vi "stop_sweep.vi"(8 "error in (no error)":errorcluster, 11 "Stimulator090724Scaffold in":refnum<class "Stimulator090724Scaffold.lvclass">) -> (0 "error out":errorcluster, 3 "Stimulator090724Scaffold out":refnum<class "Stimulator090724Scaffold.lvclass">)   [LabVIEW 2010, in "Stimulator090724Scaffold.lvclass"]
uses:
  Stimulator090724Scaffold.lvclass
  Stimulator090724Scaffold.lvclass/Stimulator090724Scaffold.ctl
  Clock/GenericClock/GenericClock/GenericClock.lvclass
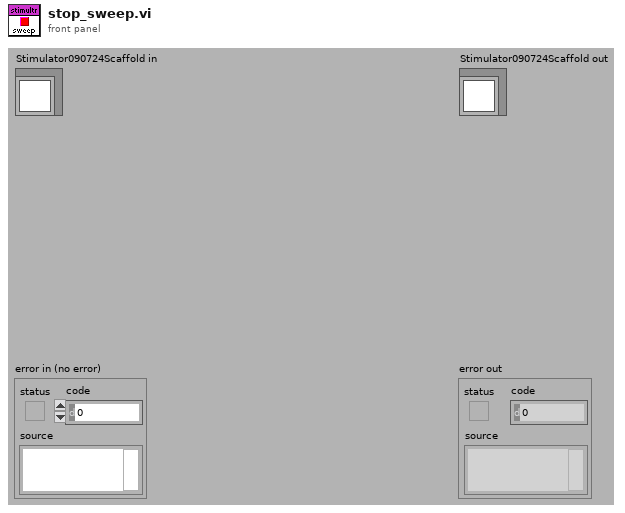
[diagram p1: front panel]
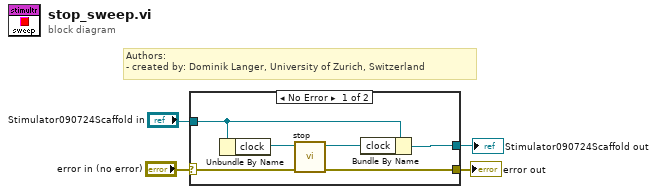
[diagram p0: block diagram]
diagram:
  # "Authors: \n- created by: Dominik Langer, University of Zurich, Switzerland"
  n1 = case shown="No Error" "error in (no error)" {
    selector: "error in (no error)" -> [w7 w12]
    tunnel: [w6 w12] -> w2
    tunnel: [w5 w11] -> w1
    tunnel: "Stimulator090724Scaffold in" -> [w9 w11]
    frame No Error {
      n2 = Unbundle By Name(w9) -> ("clock"=w10:refnum<class "GenericClock.lvclass">)
      n3 = call-dynamic "stop.vi"("error in (no error)"=w7, "GenericClock in"=w10) -> ("error out"=w6:errorcluster, "GenericClock out"=w8:refnum<class "GenericClock.lvclass">)  [unwired: 8 out]
      n4 = Bundle By Name(cluster=w9, "clock"=w8) -> (w5:refnum<class "Stimulator090724Scaffold.lvclass">)
    }
    frame Error {
    }
  }
  "error out" <- w2
  "Stimulator090724Scaffold out" <- w1
